vi "angleArray.vi"(9 "Angle step":dbl=2.5, 10 "Angle stop":dbl=60.0, 11 "Angle start":dbl=-60.0) -> (3 "Array":dbl[](array[numeric]))   [LabVIEW 2015]
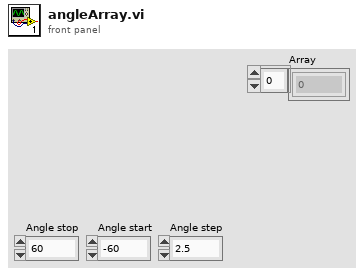
[diagram p1: front panel]
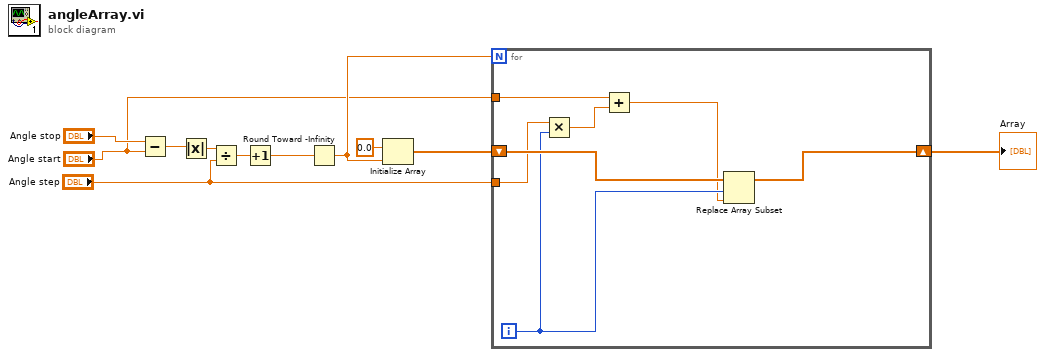
[diagram p0: block diagram]
diagram:
  n1 = Subtract(x="Angle stop", y="Angle start") -> (x-y=w10:dbl)
  n2 = Absolute Value(x=w10) -> (abs(x)=w9:dbl)
  n3 = Divide(x=w9, y="Angle step") -> (x/y=w8:dbl)
  n4 = Increment(x=w8) -> (x+1=w7:dbl)
  n5 = Round Toward -Infinity(1:w7) -> (0:w5:dbl)
  n6 = Initialize Array(0.0 ("element"), w5) -> (w4:dbl[])
  n7 = for {
    N: w5 -> [_]
    shift-right: [w17] -> w3
    shift-left: w4 -> [w18]
    tunnel: "Angle start" -> [w16]
    tunnel: "Angle step" -> [w15]
    i -> [w14]
    n8 = Multiply(x=w15, y=w14) -> (x*y=w13:dbl)
    n9 = Add(x=w16, y=w13) -> (x+y=w12:dbl)
    n10 = Replace Array Subset(array=w18, new element=w12, index=w14) -> (w17:dbl[])
  }
  "Array" <- w3
